vi "Get Position.vi"(8 "error in (no error)":errorcluster, 11 "simulated KUKA youBot arm motor in":refnum<class "NI_Robotics_KUKA youBot Arm Motor_Sim.lvclass">) -> (0 "error out":errorcluster, 2 "CCW position (rad)":dbl, 3 "simulated KUKA youBot arm motor out":refnum<class "NI_Robotics_KUKA youBot Arm Motor_Sim.lvclass">)   [LabVIEW 2017, in "NI_Robotics_KUKA youBot Host.lvlib" / "NI_Robotics_KUKA youBot Arm Motor_Sim.lvclass"]
uses:
  <vilib>/robotics/KUKA youBot/Motor/Arm Motor Sim/NI_Robotics_KUKA youBot Arm Motor_Sim.lvclass
  <vilib>/robotics/KUKA youBot/Motor/Arm Motor Sim/NI_Robotics_KUKA youBot Arm Motor_Sim.lvclass/NI_Robotics_KUKA youBot Arm Motor_Sim.ctl
  <vilib>/robotics/Simulator/Robot Factory/Motor/ODESimulator_Motor.lvclass
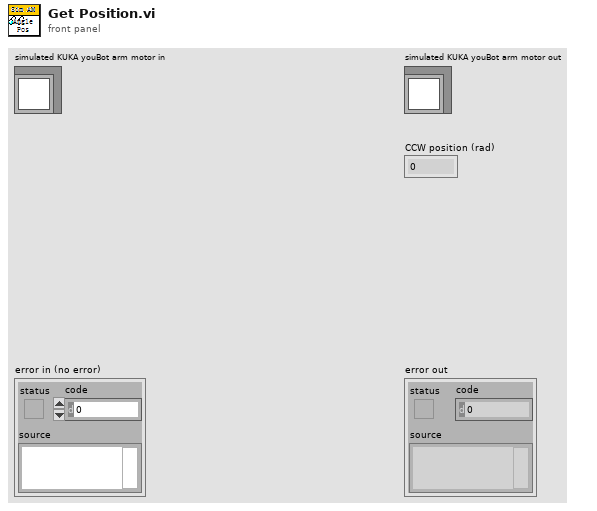
[diagram p1: front panel]
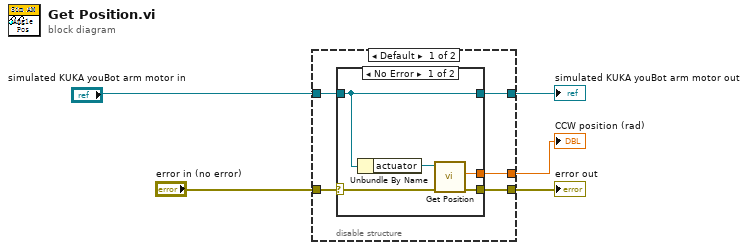
[diagram p0: block diagram]
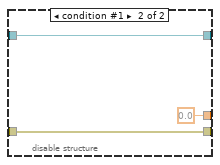
[diagram p3: hidden frame]
diagram:
  n1 = disable-structure shown="Default" {
    disable-tunnel: "simulated KUKA youBot arm motor in" -> [w10 w20]
    disable-tunnel: "error in (no error)" -> [w9 w19]
    disable-tunnel: [w8 w20] -> w3
    disable-tunnel: [w7 0.0 ("CCW Position (rad)")] -> w2
    disable-tunnel: [w6 w19] -> w1
    frame condition #0 (active) {
      n2 = case shown="No Error" w9 {
        selector: w9 -> [w13 w17]
        tunnel: [w12 w17] -> w6
        tunnel: w10 -> [w15 w16]
        tunnel: [w15 w16] -> w8
        tunnel: [w11 _] -> w7
        frame No Error {
          n3 = Unbundle By Name(w15) -> ("actuator"=w14:refnum<class "ODESimulator_Motor.lvclass">)
          n4 = call-dynamic "Get Position.vi"("error in (no error)"=w13, "Motor in"=w14) -> ("error out"=w12:errorcluster, "CCW Position (rad)"=w11:dbl)  [unwired: 7 in, 1 out]
        }
        frame Error {
        }
      }
    }
    frame condition #1 {
    }
  }
  "error out" <- w1
  "simulated KUKA youBot arm motor out" <- w3
  "CCW position (rad)" <- w2
